vi "XNET Write (State LIN Diagnostic Schedule Change).vi"(0 "session in":refnum<k21>, 5 "diagnostics schedule (null)":T1 items=["Null", "Master Request", "Slave Response"], 11 "error in (no error)":errorcluster) -> (4 "session out":refnum<k21>, 15 "error out":errorcluster)   [LabVIEW 2018]
doc: "Write a request for the LIN interface to change the diagnostic schedule. You can use this XNET Write VI with any input or output session for LIN."
uses:
  XNET LIN Diag Schedule Type.ctl
  nixlvapi.dll
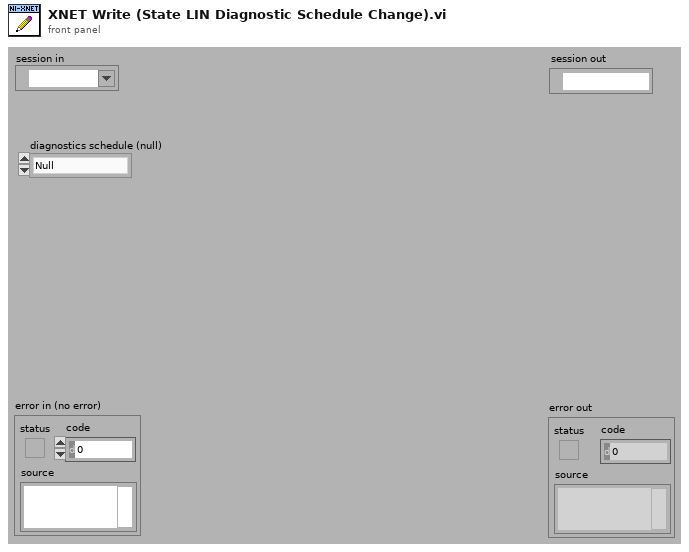
[diagram p1: front panel]
types:
  T1 = typedef "XNET LIN Diag Schedule Type.ctl" = u32
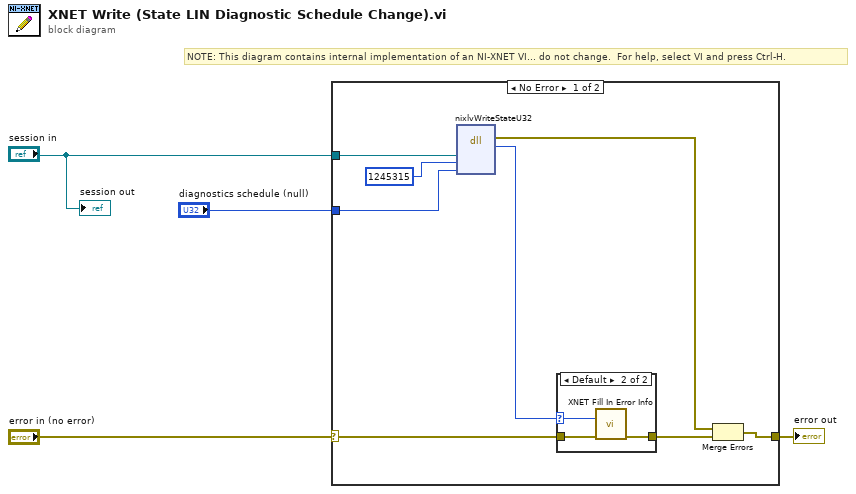
[diagram p0: block diagram]
diagram:
  # "NOTE: This diagram contains internal implementation of an NI-XNET VI... do not change.  For help, select VI and press Ctrl-H."
  n1 = case shown="No Error" "error in (no error)" {
    selector: "error in (no error)" -> [w11 w17]
    tunnel: "session in" -> [w12 _]
    tunnel: [w6 w17] -> w4
    tunnel: "diagnostics schedule (null)" -> [w7 _]
    frame No Error {
      n2 = dll-call lib="nixlvapi.*" fn="nixlvWriteStateU32"("SessionRef"=w12, "StateID"=u32 1245315, "StateValue"=w7) -> (error out=w5:errorcluster, "return type"=w9:i32)  [unwired: 5 in, 2 out]
      n3 = case shown="Default" w9 {
        selector: w9 -> [_ w14]
        tunnel: w11 -> [w13 w15]
        tunnel: [w13 w16] -> w10
        frame 0 {
        }
        frame Default {
          n4 = call "XNET Fill In Error Info.vi"("status code"=w14, "error in"=w15) -> ("error out"=w16:errorcluster)  [unwired: 13 out]
        }
      }
      n5 = Merge Errors(w5, w10) -> (w6:errorcluster)
    }
    frame Error {
    }
  }
  "error out" <- w4
  "session out" <- "session in"
